vi "Remove Malleable VIs From Library.vi"(8 "error in (no error)":errorcluster, 11 "Library Ref":refnum<vi>) -> (0 "error out":errorcluster)   [LabVIEW 2020]
doc: "Removes all of the malleable VIs from the library which were converted to polymorphic VIs."
uses:
  Global.vi
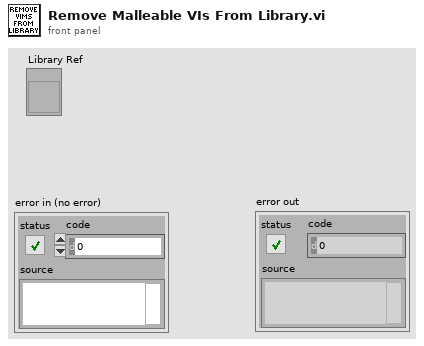
[diagram p1: front panel]
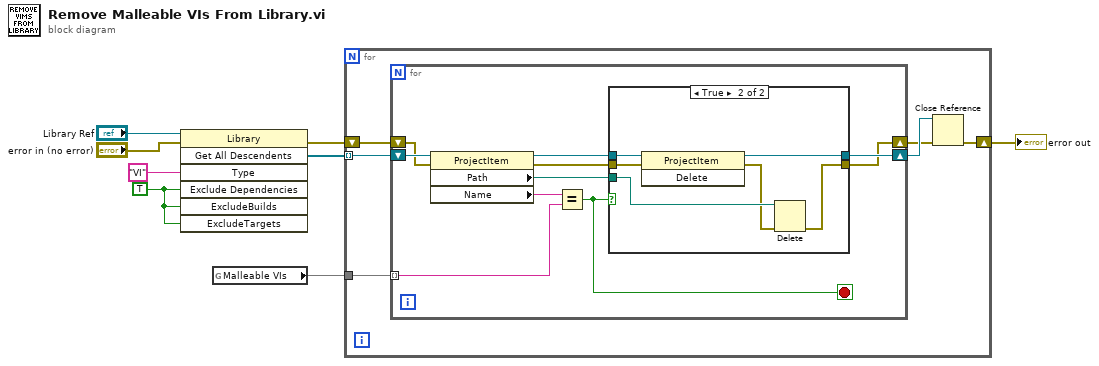
[diagram p0: block diagram]
diagram:
  w6 = TRUE ("ExcludeDependencies")
  n1 = invoke class="Library" method="Get All Descendents"(reference="Library Ref", error in="error in (no error)", "Type"="VI", "Exclude Dependencies"=w6, "ExcludeBuilds"=w6, "ExcludeTargets"=w6) -> (error out=w2:errorcluster, "All Descendents"=w5:refnum<vi>[])  [unwired: 1 in, 5 out]
  n2 = global read "Global.vi" "Malleable VIs"() -> (w4:set{string})
  n3 = for {
    tunnel: w5 -> [w14] mode=indexing
    tunnel: w4 -> [w13]
    shift-right: [w9] -> w1
    shift-left: w2 -> [w12]
    n4 = for {
      tunnel: w13 -> [w21] mode=indexing
      shift-right: [w16] -> w10
      shift-left: w12 -> [w19]
      shift-right: [w17] -> w11
      shift-left: w14 -> [w24]
      stop <- w20 stop-if-true
      n5 = property class="ProjectItem"(reference=w24, error in=w19) -> (reference out=w23:refnum<vi>, error out=w18:errorcluster, "Path"=w15:path, "Name"=w22:string)
      n6 = Equal?(x=w22, y=w21) -> (x = y?=w20:bool)
      n7 = case shown="True" w20 {
        tunnel: w23 -> [w26 w31]
        tunnel: [w26 w32] -> w17
        tunnel: w18 -> [w25 w30]
        tunnel: [w25 w28] -> w16
        tunnel: w15 -> [_ w29]
        frame False {
        }
        frame True {
          n8 = invoke class="ProjectItem" method="Delete"(reference=w31, error in=w30) -> (reference out=w32:refnum<vi>, error out=w27:errorcluster)  [unwired: 1 in, 1 out]
          n9 = Delete(path (use dialog)=w29, error in=w27) -> (error out=w28:errorcluster)  [unwired: 3 in, 2 out]
        }
      }
    }
    n10 = Close Reference(reference=w11, error in (no error)=w10) -> (error out=w9:errorcluster)
  }
  "error out" <- w1
